vi "InformationAndLog.vi"(2 "配置信息":T4, 10 "模拟数据枚举":T5(ring)) -> (14 "映射表":T2(c390), 16 "结果反馈":T3)   [LabVIEW 2019]
uses:
  <vilib>/Utility/miscctls.llb/LVMapReplaceAction.ctl
panel:
  out "数组":T1(array[ring])
  out "记录上限":dbl=200.0
  # "报文记录格式\n时间  报文分类  报文"
  # "全部原始报文输入"
  # "通讯名称（由键确认）\n记录上限\n记录格式\n通讯状态"
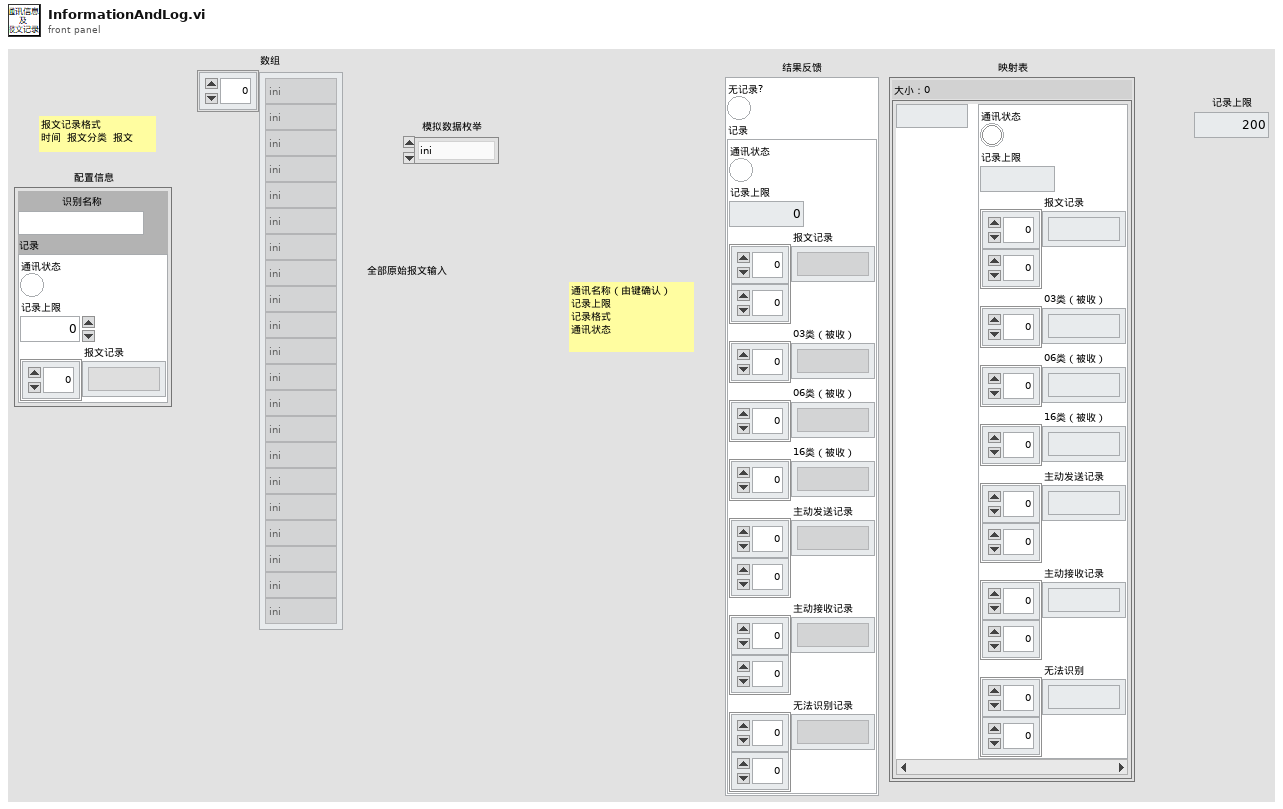
[diagram p1: front panel]
types:
  T1 = enum16{"ini", "增", "删", "查", "改-通讯状态", "改-记录上限", "增-报文", "清空报文记录", "清空全部记录"}[]
  T2 = map{string, cluster{"通讯状态":bool, "记录上限":dbl, "报文记录":string[][], "03类（被收）":string[], "06类（被收）":string[], "16类（被收）":string[], "主动发送记录":string[][], "主动接收记录":string[][], "无法识别":string[][]}}
  T3 = cluster{"无记录?":bool, "记录":cluster{"通讯状态":bool, "记录上限":dbl, "报文记录":string[][], "03类（被收）":string[], "06类（被收）":string[], "16类（被收）":string[], "主动发送记录":string[][], "主动接收记录":string[][], "无法识别记录":string[][]}}
  T4 = cluster{"识别名称":string, "记录":cluster{"通讯状态":bool, "记录上限":dbl, "报文记录":string[]}}
  T5 = enum16{"ini", "增", "删", "查", "改-通讯状态", "改-记录上限", "增-报文", "清空报文记录", "清空全部记录"}
  T6 = cluster{"通讯状态":bool, "记录上限":dbl, "报文记录":string[][], "03类（被收）":string[], "06类（被收）":string[], "16类（被收）":string[], "主动发送记录":string[][], "主动接收记录":string[][], "无法识别":string[][]}
  T7 = typedef "LVMapReplaceAction.ctl" = enum32{"Modify Entry only if found", "Add or Modify Entry", "Delete Entry"}
  T8 = cluster{"key not found?":bool, "簇":cluster{"通讯状态":bool, "记录上限":dbl, "报文记录":string[][], "03类（被收）":string[], "06类（被收）":string[], "16类（被收）":string[], "主动发送记录":string[][], "主动接收记录":string[][], "无法识别":string[][]}}
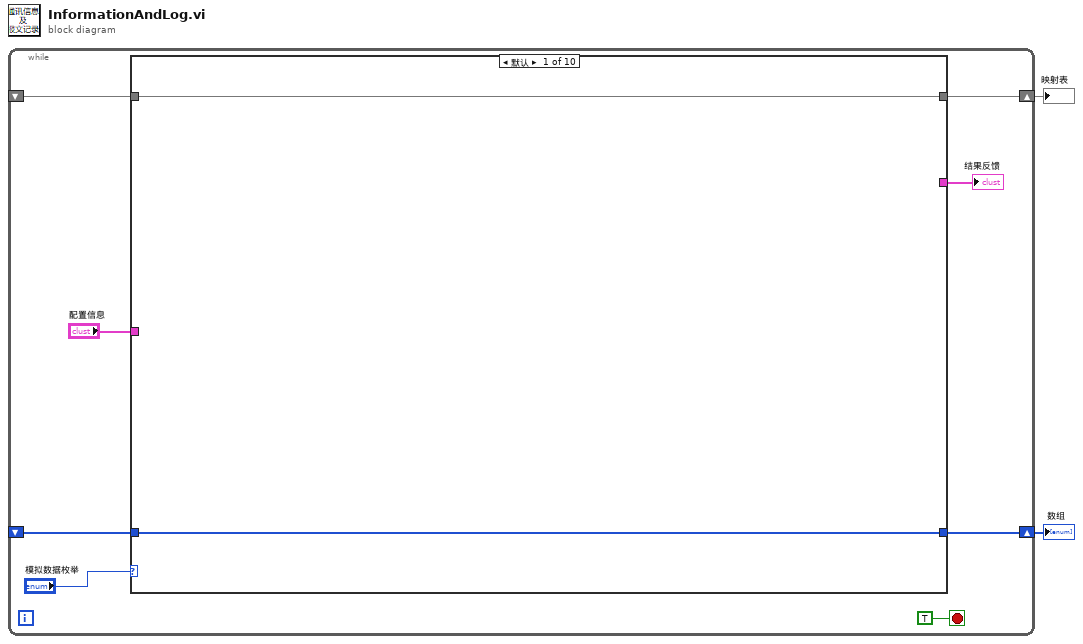
[diagram p0: block diagram]
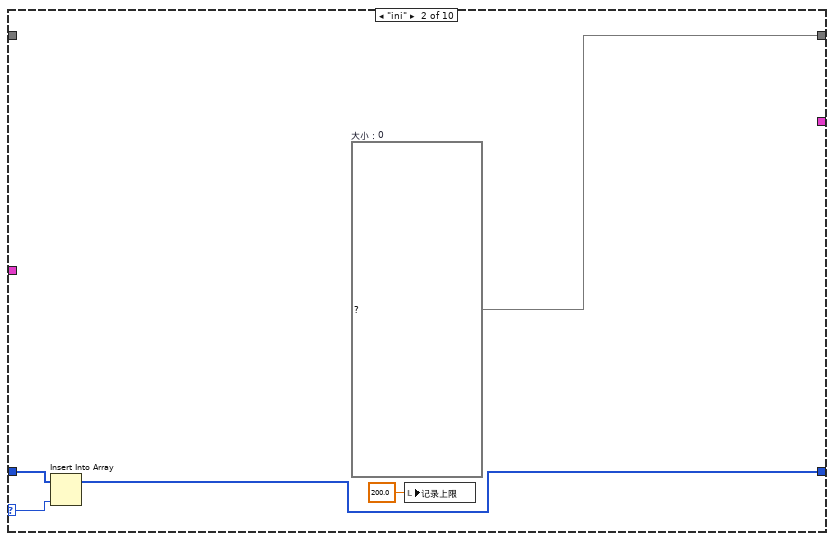
[diagram p2: hidden frame]
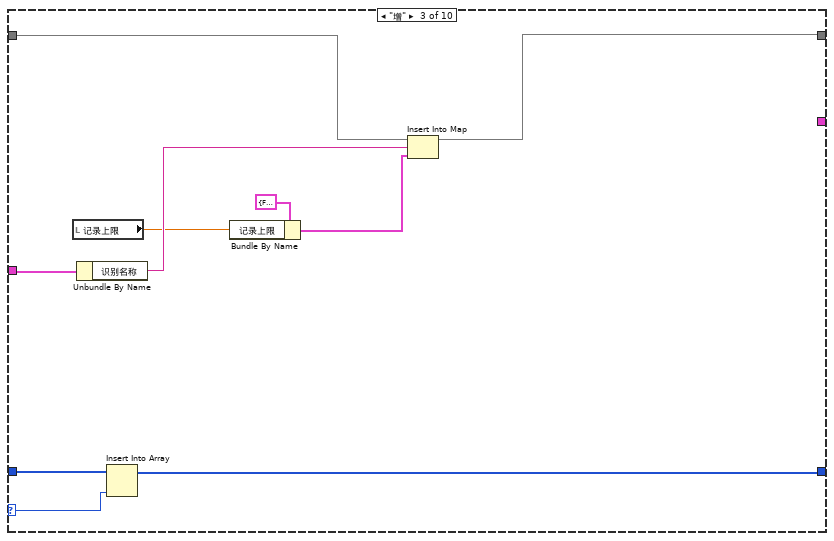
[diagram p3: hidden frame]
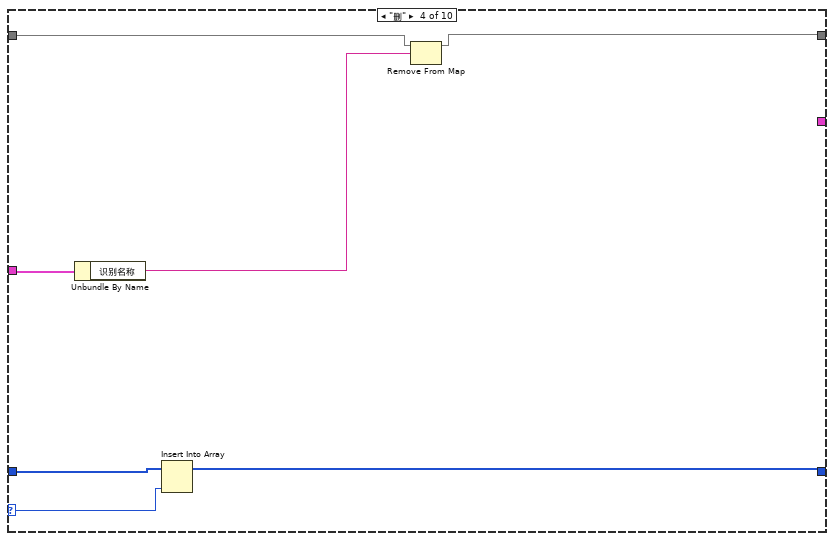
[diagram p4: hidden frame]
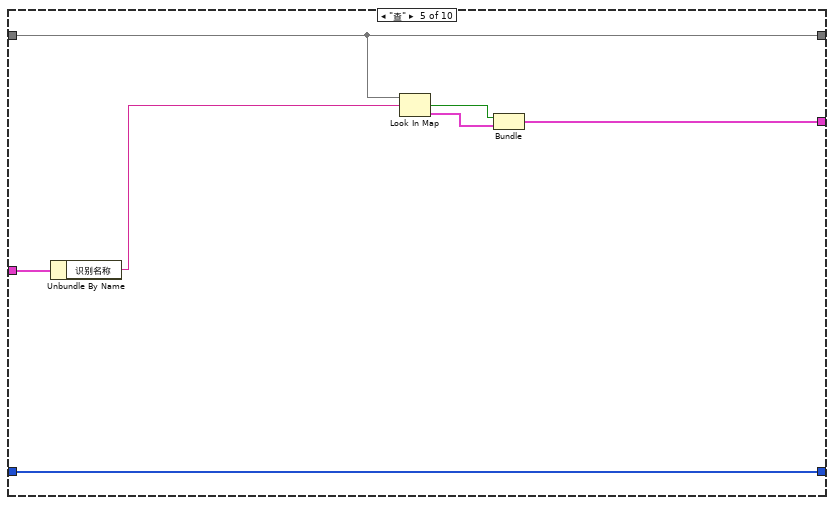
[diagram p5: hidden frame]
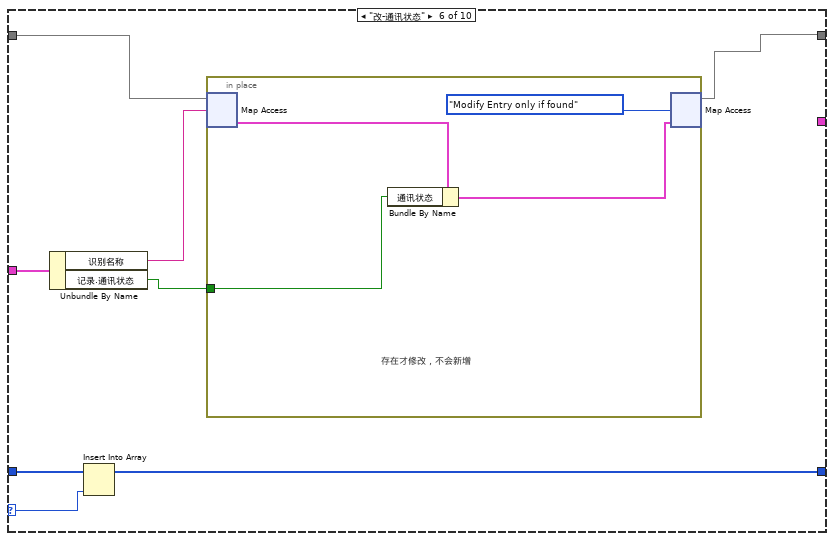
[diagram p6: hidden frame]
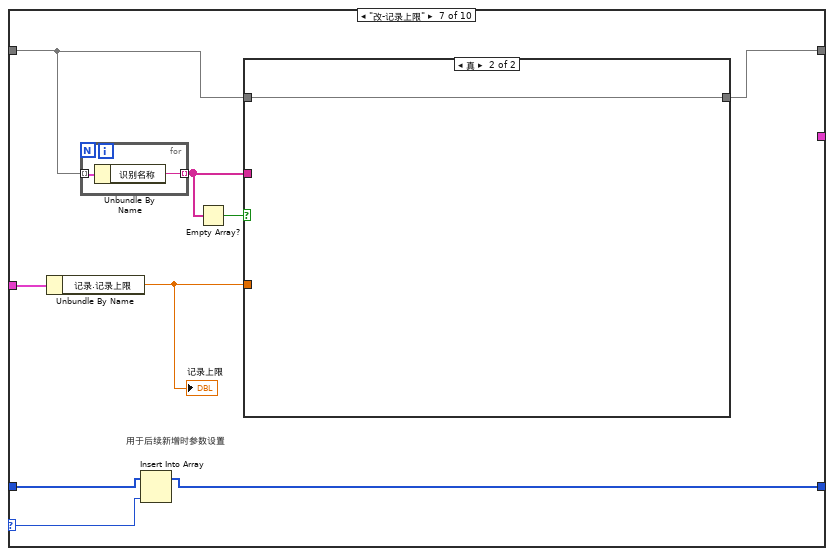
[diagram p7: hidden frame]
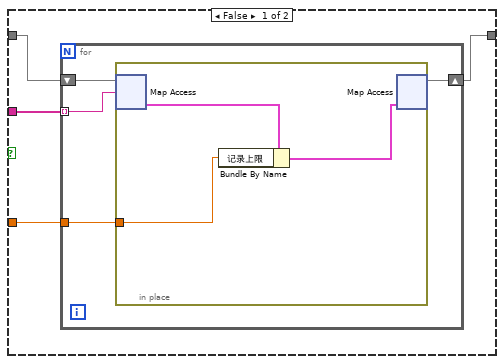
[diagram p8: hidden frame]
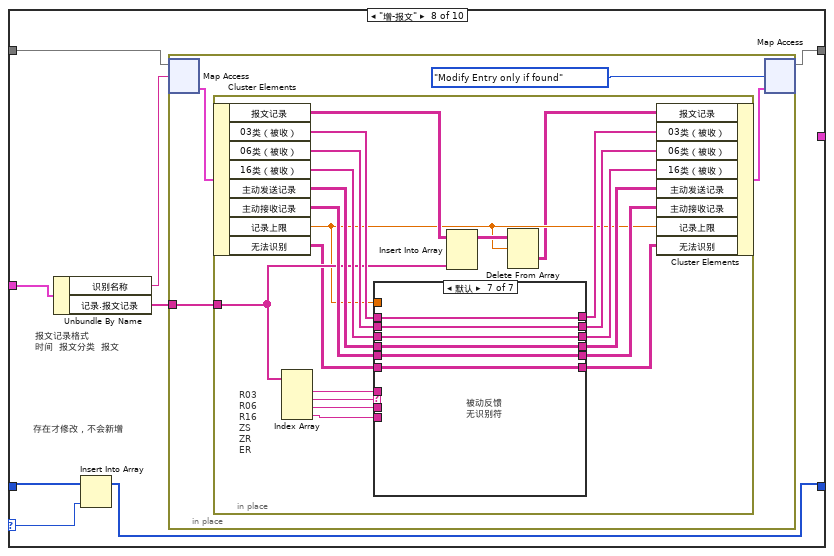
[diagram p9: hidden frame]
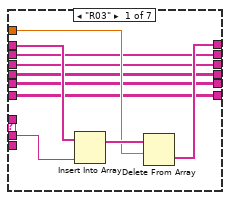
[diagram p10: hidden frame]
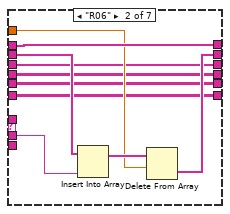
[diagram p11: hidden frame]
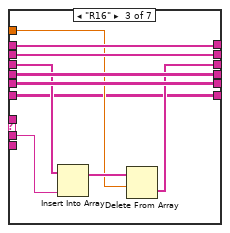
[diagram p12: hidden frame]
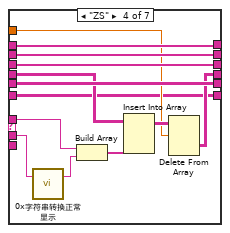
[diagram p13: hidden frame]
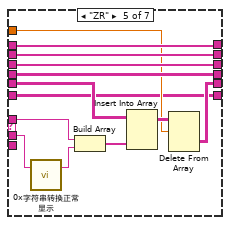
[diagram p14: hidden frame]
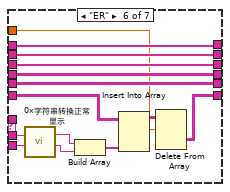
[diagram p15: hidden frame]
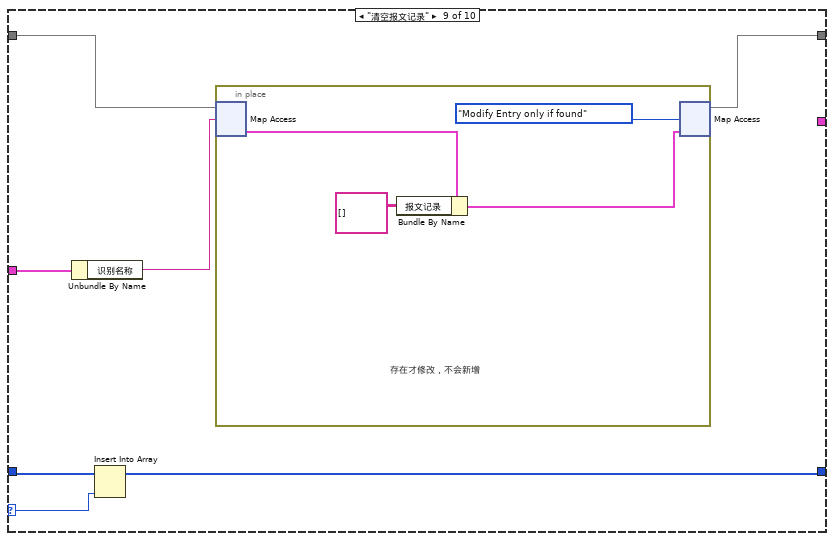
[diagram p16: hidden frame]
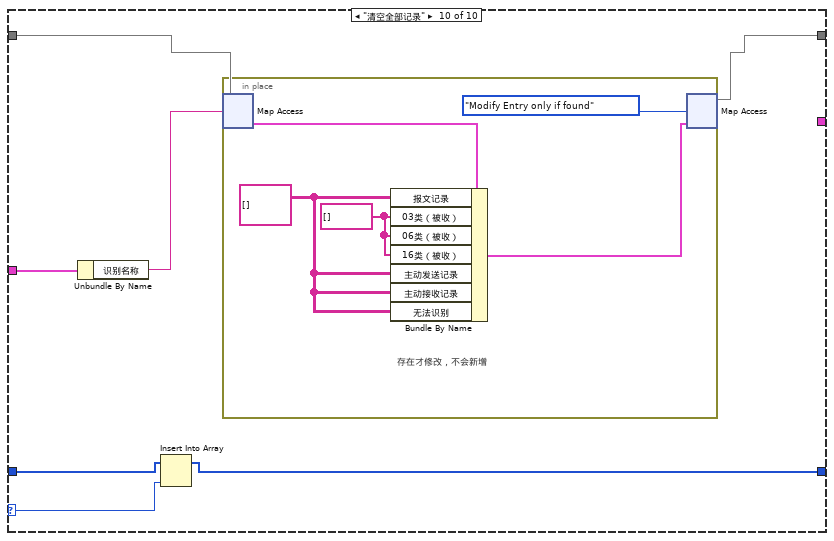
[diagram p17: hidden frame]
diagram:
  n1 = while {
    shift-right: [w6] -> w2
    shift-left: _ -> [w8]
    shift-right: [w3] -> w1
    shift-left: _ -> [w4]
    stop <- TRUE stop-if-true
    n2 = case shown="默认" "模拟数据枚举" {
      selector: "模拟数据枚举" -> [_ w14 w19 w29 _ w44 w55 w78 w186 w197]
      tunnel: w8 -> [w12 _ w27 w34 w36 w49 w61 w84 w191 w200]
      tunnel: "配置信息" -> [_ _ w26 w33 w41 w48 w62 w83 w189 w202]
      tunnel: [_ _ _ _ w37 _ _ _ _ _] -> w7
      tunnel: [w12 w16 w23 w31 w36 w45 w57 w80 w188 w199] -> w6
      tunnel: w4 -> [w11 w15 w20 w30 w35 w43 w56 w79 w187 w198]
      tunnel: [w11 w13 w18 w28 w35 w42 w54 w77 w185 w196] -> w3
      frame Default {
      }
      frame "ini" {
        w16 = T2 {}  # 大小：0
        n3 = Insert Into Array(array=w15, new element=w14) -> (w13:T1)  [unwired: 1 in]
        n4 = local write "记录上限"(200.0 ("记录上限")) -> ()
      }
      frame "增" {
        n5 = local read "记录上限"() -> (w24:dbl)
        n6 = Unbundle By Name(w26) -> ("识别名称"=w25:string)
        n7 = Insert Into Array(array=w20, new element=w19) -> (w18:T1)  [unwired: 1 in]
        n8 = Bundle By Name(cluster=T6 {"通讯状态"=FALSE, "记录上限"=0.0, "报文记录"=[], "03类（被收）"=[], "06类（被收）"=[], "16类（被收）"=[], "主动发送记录"=[], "主动接收记录"=[], "无法识别"=[]} ("值"), "记录上限"=w24) -> (w21:T6)
        n9 = Insert Into Map(map in=w27, key=w25, value=w21) -> (map out=w23:T2)  [unwired: 2 out]
      }
      frame "删" {
        n10 = Unbundle By Name(w33) -> ("识别名称"=w32:string)
        n11 = Insert Into Array(array=w30, new element=w29) -> (w28:T1)  [unwired: 1 in]
        n12 = Remove From Map(10:w32, 11:w34) -> (3:w31:T2)  [unwired: 2 out]
      }
      frame "查" {
        n13 = Unbundle By Name(w41) -> ("识别名称"=w40:string)
        n14 = Look In Map(map=w36, key=w40) -> (key not found?=w39:bool, value=w38:T6)  [unwired: 1 in]
        n15 = Bundle("key not found?"=w39, "簇"=w38) -> (w37:T8)  [unwired: 1 in]
      }
      frame "改-通讯状态" {
        n16 = Unbundle By Name(w48) -> ("识别名称"=w47:string, "记录.通讯状态"=w46:bool)
        n17 = Insert Into Array(array=w43, new element=w44) -> (w42:T1)  [unwired: 1 in]
        n18 = in-place {
          in-place-border: w46 -> [w50]
          # "存在才修改，不会新增"
          n19 = in-place-map #1(w49, w47) -> (w52:T6)  [unwired: 1 in, 1 out]
          n20 = Bundle By Name(cluster=w52, "通讯状态"=w50) -> (w51:T6)
          n21 = in-place-map #1(w51, LVMapReplaceAction."Modify Entry only if found" ("操作")) -> (w45:T2)  [unwired: 2 out]
        }
      }
      frame "改-记录上限" {
        # "用于后续新增时参数设置"
        n22 = Unbundle By Name(w62) -> ("记录.记录上限"=w58:dbl)
        "记录上限" <- w58
        n23 = for {
          tunnel: w61 -> [w76] mode=indexing
          tunnel: [w75] -> w59 mode=indexing
          n24 = Unbundle By Name(w76) -> ("识别名称"=w75:string)
        }
        n25 = Insert Into Array(array=w56, new element=w55) -> (w54:T1)  [unwired: 1 in]
        n26 = Empty Array?(array=w59) -> (empty?=w60:bool)
        n27 = case shown="真" w60 {
          tunnel: w61 -> [w66 w74]
          tunnel: [w65 w74] -> w57
          tunnel: w59 -> [w64 _]
          tunnel: w58 -> [w63 _]
          frame False {
            n28 = for {
              shift-right: [w68] -> w65
              shift-left: w66 -> [w70]
              tunnel: w64 -> [w69] mode=indexing
              tunnel: w63 -> [w67]
              n29 = in-place {
                in-place-border: w67 -> [w71]
                n30 = in-place-map #2(w70, w69) -> (w73:T6)  [unwired: 1 in, 1 out]
                n31 = Bundle By Name(cluster=w73, "记录上限"=w71) -> (w72:T6)
                n32 = in-place-map #2(w72) -> (w68:T2)  [unwired: 1 in, 2 out]
              }
            }
          }
          frame True {
          }
        }
      }
      frame "增-报文" {
        # "报文记录格式\n时间  报文分类  报文"
        # "存在才修改，不会新增"
        n33 = Unbundle By Name(w83) -> ("识别名称"=w82:string, "记录.报文记录"=w81:string[])
        n34 = Insert Into Array(array=w79, new element=w78) -> (w77:T1)  [unwired: 1 in]
        n35 = in-place {
          in-place-border: w81 -> [w86]
          n36 = in-place-map #3(w84, w82) -> (w87:T6)  [unwired: 1 in, 1 out]
          n37 = in-place {
            in-place-border: w86 -> [w96]
            # "R03\nR06\nR16\nZS\nZR\nER"
            n38 = in-place-cluster #4(w87) -> ("报文记录"=w109:string[][], "03类（被收）"=w107:string[], "06类（被收）"=w104:string[], "16类（被收）"=w103:string[], "主动发送记录"=w102:string[][], "主动接收记录"=w101:string[][], "记录上限"=w94:dbl, "无法识别"=w92:string[][])
            n39 = Index Array(array=w96) -> (element #1=w89:string, element #2=w108:string, element #3=w106:string, element #4=w90:string)  [unwired: 4 in]
            n40 = case shown="默认" w108 {
              tunnel: w107 -> [w119 w127 w139 w152 w165 w178 w184]
              tunnel: w106 -> [w118 w121 w133 w141 w154 w166 _]
              tunnel: w94 -> [w116 w126 w132 w146 w160 w172 _]
              tunnel: [w115 w127 w139 w152 w165 w178 w184] -> w105
              tunnel: w104 -> [w114 w128 w138 w151 w164 w177 w183]
              tunnel: w103 -> [w113 w124 w134 w150 w163 w176 w182]
              tunnel: w102 -> [w112 w123 w137 w147 w162 w175 w181]
              tunnel: w101 -> [w111 w122 w136 w149 w159 w174 w180]
              tunnel: [w114 w125 w138 w151 w164 w177 w183] -> w100
              tunnel: [w113 w124 w131 w150 w163 w176 w182] -> w99
              tunnel: [w112 w123 w137 w145 w162 w175 w181] -> w98
              tunnel: [w111 w122 w136 w149 w158 w174 w180] -> w97
              tunnel: w92 -> [w110 w120 w130 w144 w157 w170 w179]
              tunnel: [w110 w120 w130 w144 w157 w171 w179] -> w91
              tunnel: w90 -> [_ _ _ _ _ w169 _]
              tunnel: w89 -> [_ _ _ w143 w153 _ _]
              frame "R03" {
                n41 = Insert Into Array(array=w119, new element=w118) -> (w117:string[])  [unwired: 1 in]
                n42 = Delete From Array(array=w117, length=w116) -> (deleted portion=w115:string[])  [unwired: 1 in, 1 out]
              }
              frame "R06" {
                n43 = Insert Into Array(array=w128, new element=w121) -> (w129:string[])  [unwired: 1 in]
                n44 = Delete From Array(array=w129, length=w126) -> (deleted portion=w125:string[])  [unwired: 1 in, 1 out]
              }
              frame "R16" {
                n45 = Insert Into Array(array=w134, new element=w133) -> (w135:string[])  [unwired: 1 in]
                n46 = Delete From Array(array=w135, length=w132) -> (deleted portion=w131:string[])  [unwired: 1 in, 1 out]
              }
              frame "ZS" {
                n47 = call "0x字符串转换正常显示.vi"("普通字符串"=w141) -> ("0x普通字符串"=w140:string)  [unwired: 18 in]
                n48 = Build Array(w143, w140) -> (w142:string[])
                n49 = Insert Into Array(array=w147, new element=w142) -> (w148:string[][])  [unwired: 2 in]
                n50 = Delete From Array(array=w148, length=w146) -> (deleted portion=w145:string[][])  [unwired: 2 in, 1 out]
              }
              frame "ZR" {
                n51 = call "0x字符串转换正常显示.vi"("普通字符串"=w154) -> ("0x普通字符串"=w156:string)  [unwired: 18 in]
                n52 = Build Array(w153, w156) -> (w155:string[])
                n53 = Insert Into Array(array=w159, new element=w155) -> (w161:string[][])  [unwired: 2 in]
                n54 = Delete From Array(array=w161, length=w160) -> (deleted portion=w158:string[][])  [unwired: 2 in, 1 out]
              }
              frame "ER" {
                n55 = call "0x字符串转换正常显示.vi"("普通字符串"=w166) -> ("0x普通字符串"=w167:string)  [unwired: 18 in]
                n56 = Build Array(w167, w169) -> (w168:string[])
                n57 = Insert Into Array(array=w170, new element=w168) -> (w173:string[][])  [unwired: 2 in]
                n58 = Delete From Array(array=w173, length=w172) -> (deleted portion=w171:string[][])  [unwired: 2 in, 1 out]
              }
              frame Default {
                # "被动反馈\n无识别符"
              }
            }
            n59 = Insert Into Array(array=w109, new element=w96) -> (w95:string[][])  [unwired: 2 in]
            n60 = Delete From Array(array=w95, length=w94) -> (deleted portion=w93:string[][])  [unwired: 2 in, 1 out]
            n61 = in-place-cluster #4("报文记录"=w93, "03类（被收）"=w105, "06类（被收）"=w100, "16类（被收）"=w99, "主动发送记录"=w98, "主动接收记录"=w97, "记录上限"=w94, "无法识别"=w91) -> (w85:T6)
          }
          n62 = in-place-map #3(w85, LVMapReplaceAction."Modify Entry only if found" ("操作")) -> (w80:T2)  [unwired: 2 out]
        }
      }
      frame "清空报文记录" {
        n63 = Unbundle By Name(w189) -> ("识别名称"=w190:string)
        n64 = Insert Into Array(array=w187, new element=w186) -> (w185:T1)  [unwired: 1 in]
        n65 = in-place {
          # "存在才修改，不会新增"
          n66 = in-place-map #5(w191, w190) -> (w194:T6)  [unwired: 1 in, 1 out]
          n67 = Bundle By Name(cluster=w194, "报文记录"=string[][] []) -> (w193:T6)
          n68 = in-place-map #5(w193, LVMapReplaceAction."Modify Entry only if found" ("操作")) -> (w188:T2)  [unwired: 2 out]
        }
      }
      frame "清空全部记录" {
        n69 = Unbundle By Name(w202) -> ("识别名称"=w201:string)
        n70 = Insert Into Array(array=w198, new element=w197) -> (w196:T1)  [unwired: 1 in]
        n71 = in-place {
          w204 = string[] [] ("03类（被收）")
          w203 = string[][] [] ("报文记录")
          # "存在才修改，不会新增"
          n72 = in-place-map #6(w200, w201) -> (w206:T6)  [unwired: 1 in, 1 out]
          n73 = Bundle By Name(cluster=w206, "报文记录"=w203, "03类（被收）"=w204, "06类（被收）"=w204, "16类（被收）"=w204, "主动发送记录"=w203, "主动接收记录"=w203, "无法识别"=w203) -> (w205:T6)
          n74 = in-place-map #6(w205, LVMapReplaceAction."Modify Entry only if found" ("操作")) -> (w199:T2)  [unwired: 2 out]
        }
      }
    }
    "结果反馈" <- w7
  }
  "映射表" <- w2
  "数组" <- w1
